vi "Sweeping Turn.vi"(5 "PID gains":T1={"proportional gain (Kc)"=1.0, "integral time (Ti, min)"=0.01, "derivative time (Td, min)"=0.0} {"derivative time (Td, min)" format="%.3f"; "integral time (Ti, min)" format="%.3f"; "proportional gain (Kc)" format="%.3f"}, 6 "Target Yaw":dbl, 8 "error in":errorcluster, 9 "Acceptable Range":dbl) -> (0 "error out":errorcluster, 2 "Yaw":dbl, 3 "Yaw Output":dbl format="%.2f", 4 "Stop":bool)   [LabVIEW 2017]
uses:
  <vilib>/addons/control/pid/pid.llb/PID (DBL).vi
  <vilib>/addons/control/pid/NI_PID_pid.lvlib
panel:
  out "Target Yaw out":dbl
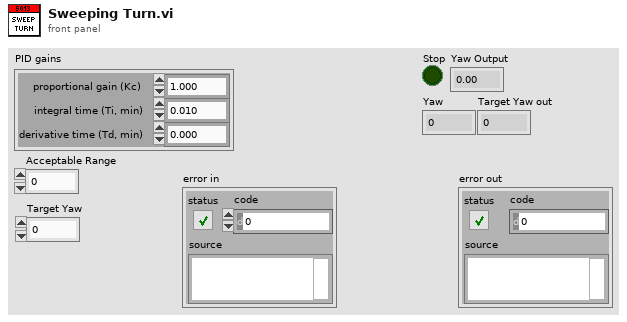
[diagram p1: front panel]
types:
  T1 = cluster{"proportional gain (Kc)":dbl, "integral time (Ti, min)":dbl, "derivative time (Td, min)":dbl}
  T2 = cluster{"Yaw":dbl, "Roll":dbl, "Pitch":dbl, "Heading":dbl, "Fused Heading":dbl}
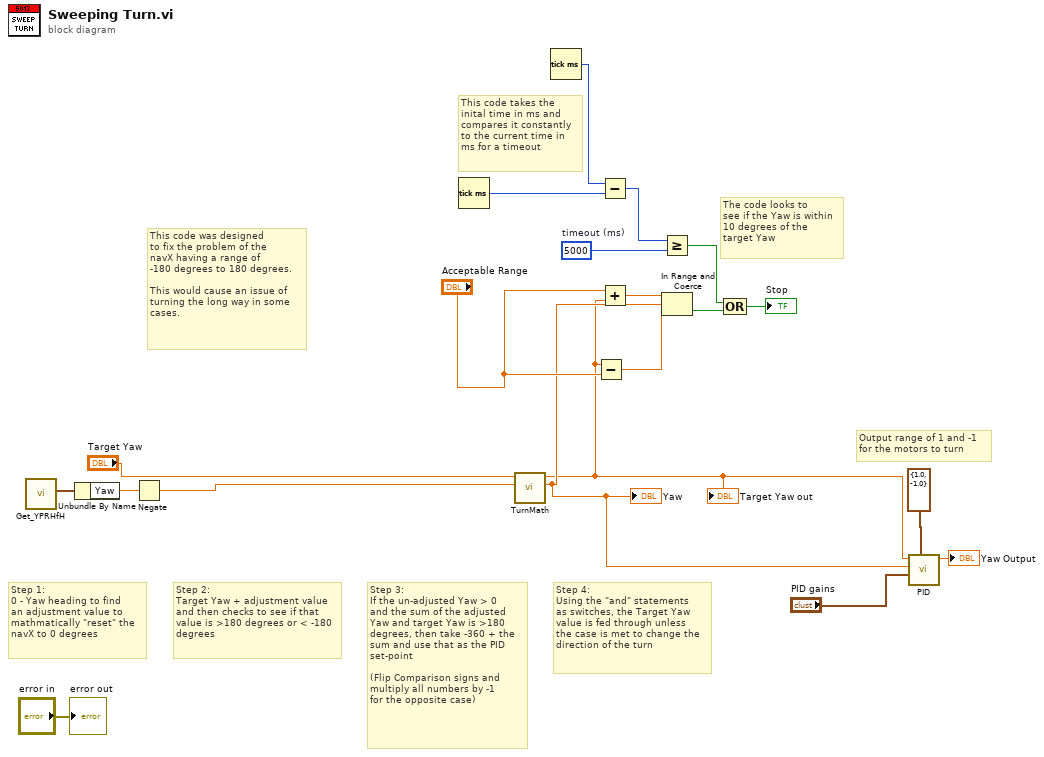
[diagram p0: block diagram]
diagram:
  w12 = u32 5000  # timeout (ms)
  # "This code was designed\nto fix the problem of the\nnavX having a range of \n-180 degrees to 180 degrees.\n\nThis would cause an issue of\nturning the long way in some\ncases."
  # "Output range of 1 and -1\nfor the motors to turn"
  # "Step 4:\nUsing the \"and\" statements\nas switches, the Target Yaw\nvalue is fed through unless\nthe case is met to change the\ndirection of the turn"
  # "Step 3:\nIf the un-adjusted Yaw > 0 \nand the sum of the adjusted \nYaw and target Yaw is >180\ndegrees, then take -360 + the \nsum and use that as the PID \nset-point\n\n(Flip Comparison signs and\nmultiply all numbers by -1 \nfor the opposite case)"
  # "Step 2:\nTarget Yaw + adjustment value\nand then checks to see if that \nvalue is >180 degrees or < -180\ndegrees"
  # "Step 1: \n0 - Yaw heading to find\nan adjustment value to \nmathmatically \"reset\" the\nnavX to 0 degrees"
  # "The code looks to \nsee if the Yaw is within\n10 degrees of the \ntarget Yaw"
  # "This code takes the\ninital time in ms and\ncompares it constantly\nto the current time in\nms for a timeout"
  n1 = call <vilib>:"Get_YPRHfH.vi"() -> ("YRPHfH"=w5:T2)  [unwired: 11 in]
  n2 = Unbundle By Name(w5) -> ("Yaw"=w4:dbl)
  n3 = Negate(x=w4) -> (-x=w3:dbl)
  n4 = Tick Count (ms)() -> (millisecond timer value=w19:u32)
  n5 = call "TurnMath.vi"("Yaw in"=w3, "Target Yaw in"="Target Yaw") -> ("Yaw out"=w2:dbl, "Target Yaw out"=w1:dbl)  [unwired: 8 in]
  "Yaw" <- w2
  "Target Yaw out" <- w1
  n6 = Tick Count (ms)() -> (millisecond timer value=w16:u32)
  n7 = Subtract(x=w1, y="Acceptable Range") -> (x-y=w10:dbl)
  n8 = Subtract(x=w16, y=w19) -> (x-y=w15:u32)
  n9 = Add(x="Acceptable Range", y=w1) -> (x+y=w9:dbl)
  n10 = Greater Or Equal?(x=w15, y=w12) -> (x >= y?=w13:bool)
  n11 = In Range and Coerce(upper limit=w9, x=w2, lower limit=w10) -> (In Range?=w11:bool)  [unwired: 1 out]
  n12 = Compound Arithmetic op=OR(w13, w11) -> (→"Stop":bool)
  n13 = call-poly <vilib>:"PID.vi"("output range"=cluster{"output high":dbl, "output low":dbl} {"output high"=1.0, "output low"=-1.0}, "PID gains"="PID gains", "process variable"=w2, "setpoint"=w1) -> ("output"=→"Yaw Output":dbl)  [unwired: 6 in, 1 out]
  "error out" <- "error in"
